vi "lookupElement.vi"(6 "typeEnum":T1(ring)=enum."xmlNode", 8 "error in (no error)":errorcluster, 9 "serachElement":string, 10 "searchInElement":string, 11 "SettingsManager in":refnum<class "SettingsManager.lvclass">) -> (0 "error out":errorcluster, 1 "returnedElements":string, 3 "SettingsManager out":refnum<class "SettingsManager.lvclass">)   [LabVIEW 2011, in "Tools.lvlib" / "Settings.lvlib" / "SettingsManager.lvclass"]
uses:
  SettingsManager.lvclass
  SettingsManager.lvclass/SettingsManager.ctl
  xmlNode/xmlNode.lvclass
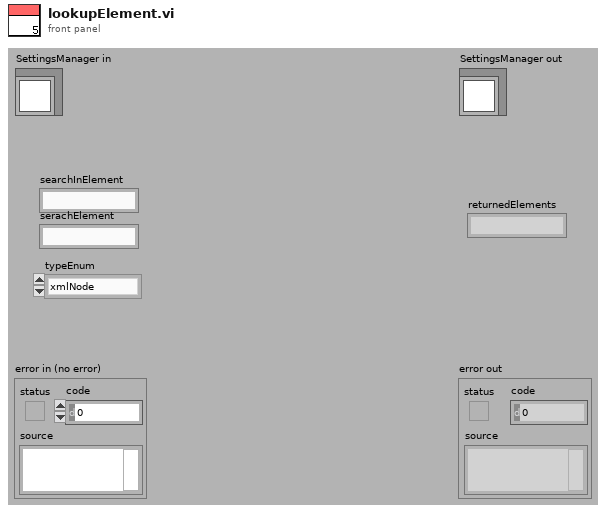
[diagram p1: front panel]
types:
  T1 = enum16{"Number", "String", "NumberArray", "StringArray", "xmlNode"}
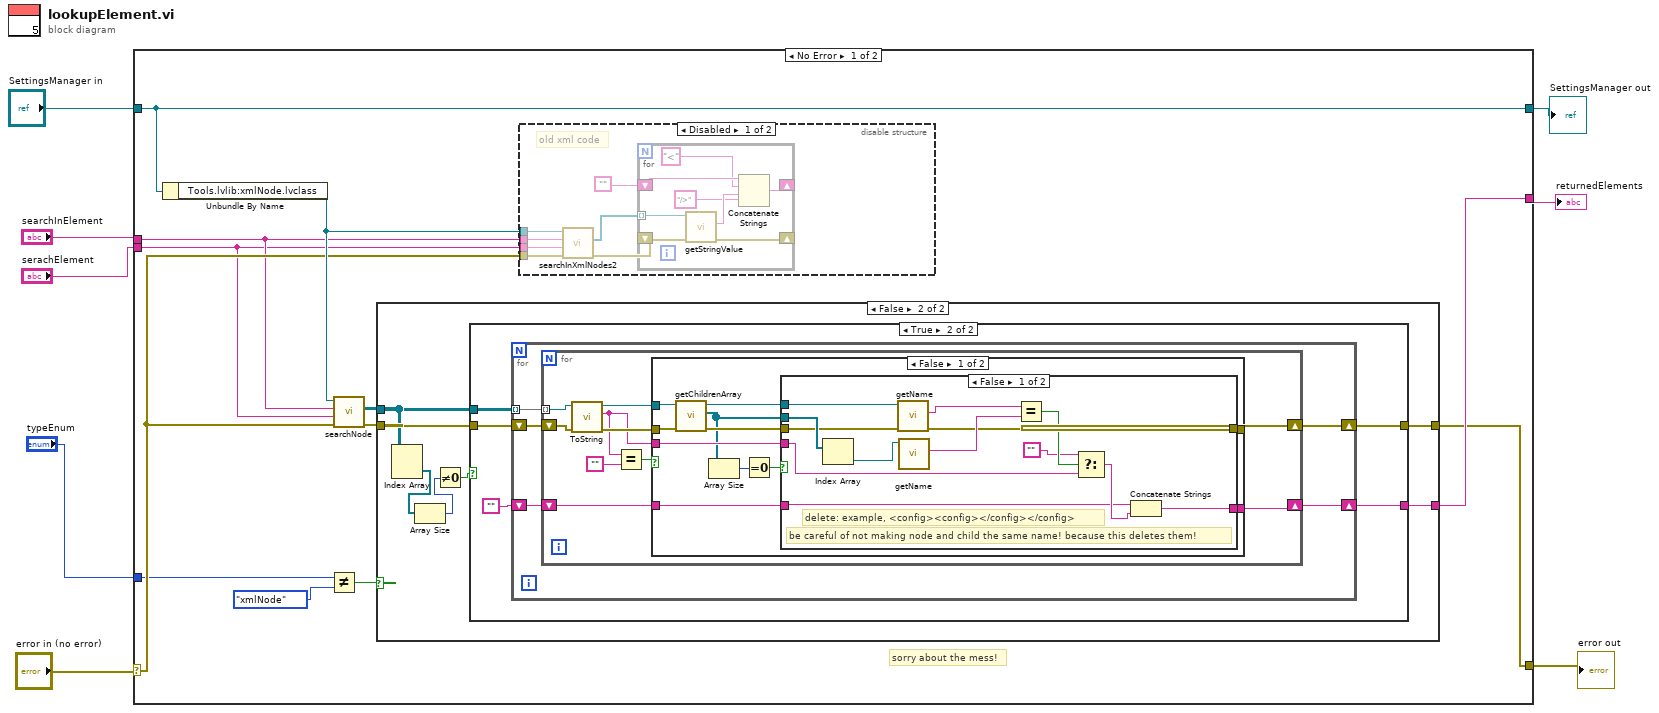
[diagram p0: block diagram]
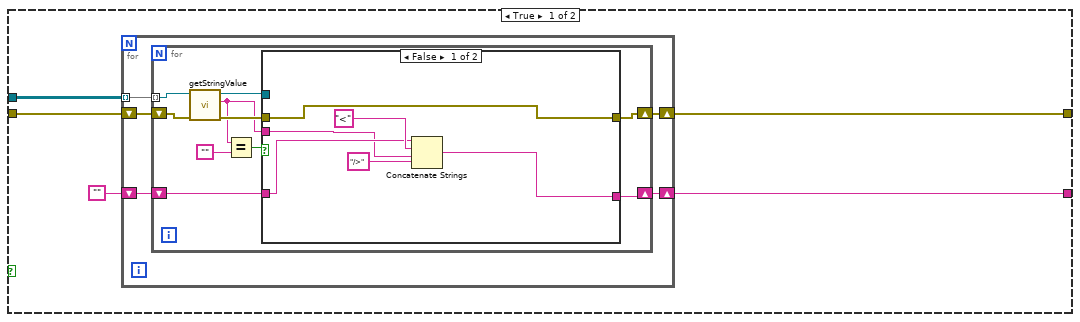
[diagram p2: hidden frame]
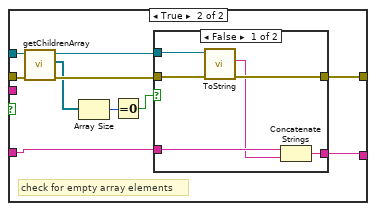
[diagram p3: hidden frame]
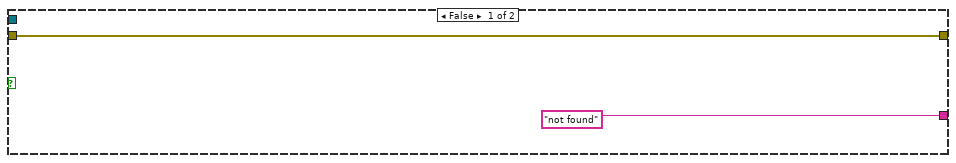
[diagram p5: hidden frame]
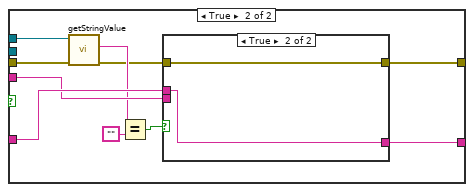
[diagram p6: hidden frame]
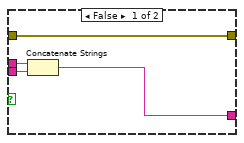
[diagram p7: hidden frame]
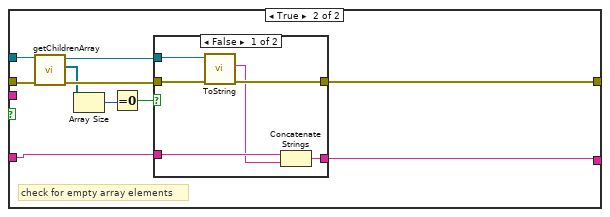
[diagram p8: hidden frame]
diagram:
  n1 = case shown="No Error" "error in (no error)" {
    selector: "error in (no error)" -> [w18 w168]
    tunnel: [w12 w168] -> w7
    tunnel: [w20 w167] -> w5
    tunnel: "SettingsManager in" -> [w20 w167]
    tunnel: "searchInElement" -> [w15 _]
    tunnel: "serachElement" -> [w14 _]
    tunnel: [w13 _] -> w2
    tunnel: "typeEnum" -> [w10 _]
    frame No Error {
      # "sorry about the mess!"
      n2 = Unbundle By Name(w20) -> ("Tools.lvlib:xmlNode.lvclass"=w19:refnum<class "xmlNode.lvclass">)
      n3 = Not Equal?(x=w10, y=T1."xmlNode" ("typeEnum")) -> (x != y?=w11:bool)
      n4 = call-dynamic "searchNode.vi"("error in (no error)"=w18, "searchElementName"=w14, "searchElementIn"=w15, "xmlNode in"=w19) -> ("error out"=w16:errorcluster, "arrayXmlNodes"=w17:refnum<class "xmlNode.lvclass">[][])  [unwired: 5 in, 1 out]
      n5 = case shown="False" w11 {
        tunnel: w17 -> [w25 w66]
        tunnel: w16 -> [w24 w71]
        tunnel: [w22 w70] -> w13
        tunnel: [w21 w69] -> w12
        frame True {
          n6 = for {
            tunnel: w25 -> [w30] mode=indexing
            shift-right: [w28] -> w21
            shift-left: w24 -> [w29]
            shift-right: [w26] -> w22
            shift-left: "" -> [w27]
            n7 = for {
              tunnel: w30 -> [w40] mode=indexing
              shift-right: [w37] -> w28
              shift-left: w29 -> [w39]
              shift-right: [w32] -> w26
              shift-left: w27 -> [w33]
              n8 = call-dynamic "getStringValue.vi"("error in (no error)"=w39, "xmlNode.lvclass in"=w40) -> ("error out"=w38:errorcluster, "stringValue"=w31:string, "xmlNode.lvclass out"=w34:refnum<class "xmlNode.lvclass">)  [unwired: 7 in]
              n9 = Equal?(x=w31, y="") -> (x = y?=w36:bool)
              n10 = case shown="False" w36 {
                tunnel: w38 -> [w41 w52]
                tunnel: [w41 w56] -> w37
                tunnel: w34 -> [_ w53]
                tunnel: w33 -> [w44 w55]
                tunnel: [w42 w54] -> w32
                tunnel: w31 -> [w43 _]
                frame False {
                  n11 = Concatenate Strings(w44, "<", w43, "/>") -> (w42:string)
                }
                frame True {
                  # "check for empty array elements"
                  n12 = call-dynamic "getChildrenArray.vi"("error in (no error)"=w52, "xmlNode.lvclass in"=w53) -> ("error out"=w51:errorcluster, "Children"=w49:refnum<class "xmlNode.lvclass">[], "xmlNode.lvclass out"=w50:refnum<class "xmlNode.lvclass">)  [unwired: 7 in]
                  n13 = Array Size(array=w49) -> (size(s)=w48:i32)
                  n14 = Equal To 0?(x=w48) -> (x = 0?=w47:bool)
                  n15 = case shown="False" w47 {
                    tunnel: w50 -> [w62 _]
                    tunnel: w51 -> [w61 w63]
                    tunnel: [w60 w63] -> w56
                    tunnel: w55 -> [w59 w64]
                    tunnel: [w57 w64] -> w54
                    frame False {
                      n16 = call-dynamic "ToString.vi"("error in (no error)"=w61, "xmlNode in"=w62) -> ("error out"=w60:errorcluster, "xml"=w58:string)  [unwired: 7 in, 1 out]
                      n17 = Concatenate Strings(w59, w58) -> (w57:string)
                    }
                    frame True {
                    }
                  }
                }
              }
            }
          }
        }
        frame False {
          n18 = Index Array(array=w66) -> (element=w65:refnum<class "xmlNode.lvclass">[])  [unwired: 2 in]
          n19 = Array Size(array=w65) -> (size(s)=w67:i32)
          n20 = Not Equal To 0?(x=w67) -> (x != 0?=w68:bool)
          n21 = case shown="True" w68 {
            tunnel: w71 -> [w72 w78]
            tunnel: ["not found" w76] -> w70
            tunnel: [w72 w75] -> w69
            tunnel: w66 -> [_ w74]
            frame False {
            }
            frame True {
              n22 = for {
                tunnel: w74 -> [w83] mode=indexing
                shift-right: [w81] -> w75
                shift-left: w78 -> [w82]
                shift-right: [w79] -> w76
                shift-left: "" -> [w80]
                n23 = for {
                  tunnel: w83 -> [w87] mode=indexing
                  shift-right: [w93] -> w81
                  shift-left: w82 -> [w88]
                  shift-right: [w89] -> w79
                  shift-left: w80 -> [w90]
                  n24 = call-dynamic "ToString.vi"("error in (no error)"=w88, "xmlNode in"=w87) -> ("error out"=w85:errorcluster, "xml"=w84:string, "xmlNode out"=w86:refnum<class "xmlNode.lvclass">)  [unwired: 7 in]
                  n25 = Equal?(x=w84, y="") -> (x = y?=w92:bool)
                  n26 = case shown="False" w92 {
                    tunnel: w85 -> [w99 w140]
                    tunnel: [w101 w143] -> w93
                    tunnel: w90 -> [w104 w142]
                    tunnel: [w103 w141] -> w89
                    tunnel: w84 -> [w102 _]
                    tunnel: w86 -> [w100 w134]
                    frame False {
                      n27 = call-dynamic "getChildrenArray.vi"("error in (no error)"=w99, "xmlNode.lvclass in"=w100) -> ("error out"=w97:errorcluster, "Children"=w94:refnum<class "xmlNode.lvclass">[], "xmlNode.lvclass out"=w98:refnum<class "xmlNode.lvclass">)  [unwired: 7 in]
                      n28 = Array Size(array=w94) -> (size(s)=w96:i32)
                      n29 = Equal To 0?(x=w96) -> (x = 0?=w95:bool)
                      n30 = case shown="False" w95 {
                        tunnel: w104 -> [w112 w127]
                        tunnel: [w117 w126] -> w103
                        tunnel: w102 -> [w111 w125]
                        tunnel: [w105 w120] -> w101
                        tunnel: w98 -> [w109 w119]
                        tunnel: w97 -> [w110 w118]
                        tunnel: w94 -> [w116 _]
                        frame False {
                          # "be careful of not making node and child the same name! because this deletes them!"
                          # "delete: example, <config><config></config></config>"
                          n31 = Index Array(array=w116) -> (element=w107:refnum<class "xmlNode.lvclass">)  [unwired: 1 in]
                          n32 = call-dynamic "getName.vi"("error in (no error)"=w110, "xmlNode.lvclass in"=w109) -> ("error out"=w105:errorcluster, "name"=w108:string)  [unwired: 7 in, 1 out]
                          n33 = call-dynamic "getName.vi"("xmlNode.lvclass in"=w107) -> ("name"=w106:string)  [unwired: 8 in, 2 out]
                          n34 = Equal?(x=w108, y=w106) -> (x = y?=w115:bool)
                          n35 = Select(t="", s=w115, f=w111) -> (s? t:f=w113:string)
                          n36 = Concatenate Strings(w112, w113) -> (w117:string)
                        }
                        frame True {
                          n37 = call-dynamic "getStringValue.vi"("error in (no error)"=w118, "xmlNode.lvclass in"=w119) -> ("error out"=w121:errorcluster, "stringValue"=w122:string)  [unwired: 7 in, 1 out]
                          n38 = Equal?(x=w122, y="") -> (x = y?=w123:bool)
                          n39 = case shown="True" w123 {
                            tunnel: w127 -> [w131 w133]
                            tunnel: [w130 w133] -> w126
                            tunnel: w125 -> [w129 _]
                            tunnel: w121 -> [w128 w132]
                            tunnel: [w128 w132] -> w120
                            frame False {
                              n40 = Concatenate Strings(w131, w129) -> (w130:string)
                            }
                            frame True {
                            }
                          }
                        }
                      }
                    }
                    frame True {
                      # "check for empty array elements"
                      n41 = call-dynamic "getChildrenArray.vi"("error in (no error)"=w140, "xmlNode.lvclass in"=w134) -> ("error out"=w139:errorcluster, "Children"=w137:refnum<class "xmlNode.lvclass">[], "xmlNode.lvclass out"=w138:refnum<class "xmlNode.lvclass">)  [unwired: 7 in]
                      n42 = Array Size(array=w137) -> (size(s)=w136:i32)
                      n43 = Equal To 0?(x=w136) -> (x = 0?=w135:bool)
                      n44 = case shown="False" w135 {
                        tunnel: w138 -> [w149 _]
                        tunnel: w139 -> [w148 w150]
                        tunnel: [w147 w150] -> w143
                        tunnel: w142 -> [w146 w151]
                        tunnel: [w144 w151] -> w141
                        frame False {
                          n45 = call-dynamic "ToString.vi"("error in (no error)"=w148, "xmlNode in"=w149) -> ("error out"=w147:errorcluster, "xml"=w145:string)  [unwired: 7 in, 1 out]
                          n46 = Concatenate Strings(w146, w145) -> (w144:string)
                        }
                        frame True {
                        }
                      }
                    }
                  }
                }
              }
            }
          }
        }
      }
      n47 = disable-structure shown="Disabled" {
        disable-tunnel: w19 -> [w156 _]
        disable-tunnel: w18 -> [w155 _]
        disable-tunnel: w15 -> [w154 _]
        disable-tunnel: w14 -> [w153 _]
        frame Disabled {
          # "old xml code"
          n48 = call-dynamic "searchInXmlNodes2.vi"("error in (no error)"=w155, "searchElementName"=w153, "searchElementIn"=w154, "xmlNode in"=w156) -> ("error out"=w157:errorcluster, "arrayXmlNodes"=w152:refnum<class "xmlNode.lvclass">[])  [unwired: 5 in, 1 out]
          n49 = for {
            shift-right: [w164] -> _
            shift-left: "" -> [w163]
            tunnel: w152 -> [w166] mode=indexing
            shift-right: [w160] -> _
            shift-left: w157 -> [w165]
            n50 = call-dynamic "getStringValue.vi"("error in (no error)"=w165, "xmlNode.lvclass in"=w166) -> ("error out"=w160:errorcluster, "stringValue"=w161:string)  [unwired: 7 in, 1 out]
            n51 = Concatenate Strings(w163, "<", w161, "/>") -> (w164:string)
          }
        }
        frame Enabled {
        }
      }
    }
    frame Error {
    }
  }
  "error out" <- w7
  "SettingsManager out" <- w5
  "returnedElements" <- w2
